vi "Read Anything INI Tag Lookup.vi"(10 "Str":string, 11 "State In":T1={"StrToSpecifiedText"=variant, "Specified Data"=variant, "Options"={"TimeStamp Format"="", "Integer format"=""}, "FloatFormat"="%#_13g"}) -> (1 "INI Text":string, 2 "Text Found?":bool, 3 "State Out":T1={"StrToSpecifiedText"=variant, "Specified Data"=variant, "Options"={"TimeStamp Format"="", "Integer format"=""}, "FloatFormat"="%#_13g"})   [LabVIEW 2020]
doc: "Look for the specified tag in the Read Anything File. If not found, the tag is looked for in the Default Data of the variant.\n\nFreeware from Moore Good Ideas, inc: www.MooreGoodIdeas.com. Do not remove this line."
uses:
  Read Write Tag Lookup Cluster.ctl
  Read Write Options Cluster.ctl
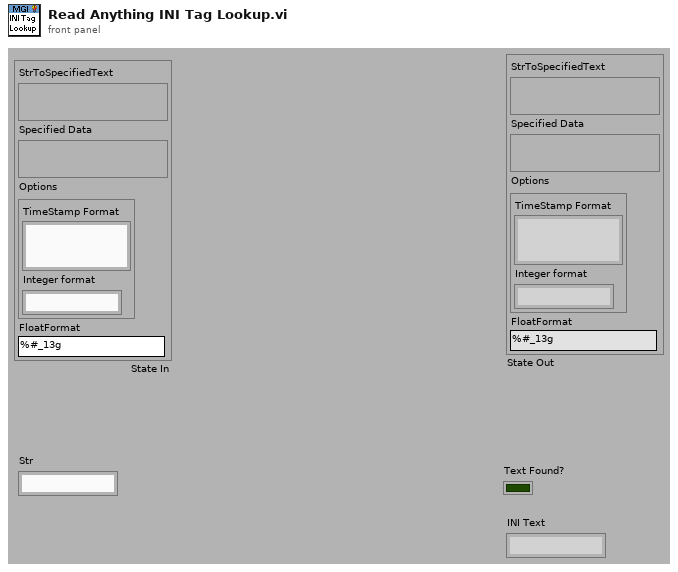
[diagram p1: front panel]
types:
  T1 = typedef "Read Write Tag Lookup Cluster.ctl" = cluster{"StrToSpecifiedText":variant, "Specified Data":variant, "Options":T2, "FloatFormat":string}
  T2 = typedef "Read Write Options Cluster.ctl" = cluster{"TimeStamp Format":string, "Integer format":string}
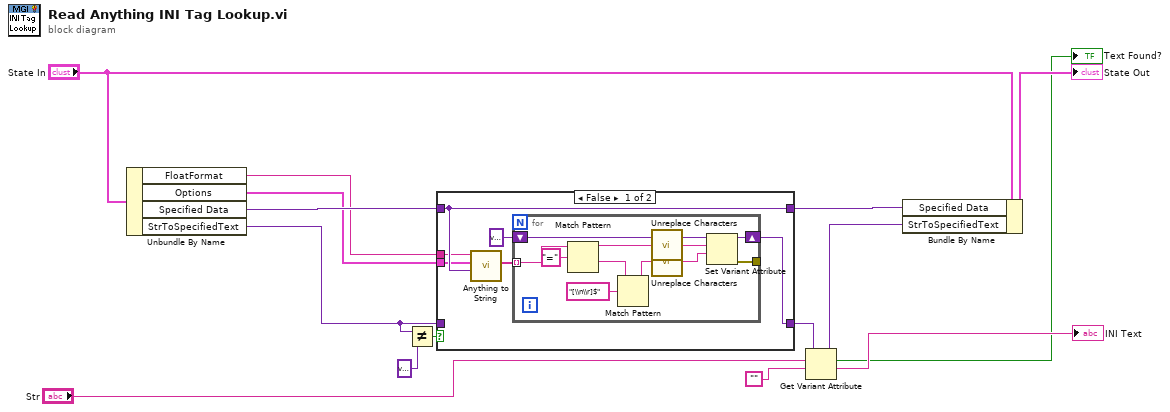
[diagram p0: block diagram]
diagram:
  n1 = Unbundle By Name("State In") -> ("FloatFormat"=w8:string, "Options"=w7:T2, "Specified Data"=w11:variant, "StrToSpecifiedText"=w2:variant)
  n2 = Not Equal?(x=w2, y=variant ("StrToDefault Variant")) -> (x != y?=w5:bool)
  n3 = case shown="False" w5 {
    tunnel: w2 -> [_ w33]
    tunnel: w11 -> [w21 w34]
    tunnel: [w21 w34] -> w10
    tunnel: [w19 w33] -> w4
    tunnel: w8 -> [w17 _]
    tunnel: w7 -> [w16 _]
    frame False {
      n4 = call "Anything to String.vi"("Anything"=w21, "Read/Write Options"=w16, "Format String (%#_13g)"=w17) -> ("Strings[]"=w18:string[])  [unwired: 1 in, 7 out]
      n5 = for {
        shift-right: [w30] -> w19
        shift-left: variant ("variant") -> [w31]
        tunnel: w18 -> [w26] mode=indexing
        tunnel: [w25] -> _
        n6 = Match Pattern(string=w26, regular expression="=") -> (before substring=w29:string, after substring=w24:string)  [unwired: 3 out]
        n7 = Match Pattern(string=w24, regular expression="[\\n\\r]$") -> (before substring=w23:string)  [unwired: 4 out]
        n8 = call "Unreplace Characters.vi"("String In"=w29) -> ("String Out"=w28:string)  [unwired: 1 out]
        n9 = call "Unreplace Characters.vi"("String In"=w23) -> ("String Out"=w27:string)  [unwired: 1 out]
        n10 = Set Variant Attribute(Variant=w31, name=w28, value=w27) -> (Variant out=w30:variant, error out=w25:errorcluster)  [unwired: 1 in, 1 out]
      }
    }
    frame True {
    }
  }
  n11 = Get Variant Attribute(Variant=w4, name="Str", default value (empty Variant)="") -> (duplicate Variant=w1:variant, found=→"Text Found?":bool, value=→"INI Text":string)  [unwired: 1 in, 1 out]
  n12 = Bundle By Name(cluster="State In", "Specified Data"=w10, "StrToSpecifiedText"=w1) -> (→"State Out":T1)
